vi "Calculate Particle Scores.vi"(7 "Pixel Value":i32=1, 8 "Limit Tests?":bool=TRUE, 9 "Aspect Fudge Factor":dbl=1.0, 10 "Sorted Data":dbl[][](array[numeric]), 11 "Image in":T2) -> (3 "Scores":T1(array[cluster]))   [LabVIEW 2015]
doc: "Calculate scores based on the particle measurements. Calculated scores are for aspect ratio, area to convex hull area, masking, and moment of inertia. These scores range between 0 and 100 and can be used to categorize particles as targets and non-targets. The fudge factor compensates for camera modes that do not give square pixels."
uses:
  <vilib>/vision/Image Controls.llb/IMAQ Image.ctl
  <vilib>/vision/NI_Vision_Development_Module.lvlib
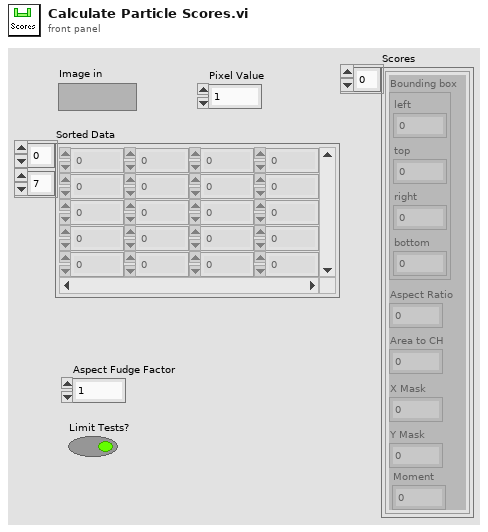
[diagram p1: front panel]
types:
  T1 = cluster{"Bounding box":cluster{"left":dbl, "top":dbl, "right":dbl, "bottom":dbl}, "Aspect Ratio":dbl, "Area to CH":dbl, "X Mask":dbl, "Y Mask":dbl, "Moment":dbl}[]
  T2 = typedef "IMAQ Image.ctl" = refnum<image>
  T3 = cluster{"[0]":dbl, "[1]":dbl, "[2]":dbl, "[3]":dbl}
  T4 = cluster{cluster{"[0]":dbl, "[1]":dbl, "[2]":dbl, "[3]":dbl}, "Aspect Ratio Score":dbl, "Score":dbl, "X Score":dbl, "Y Score":dbl, "Score":dbl}
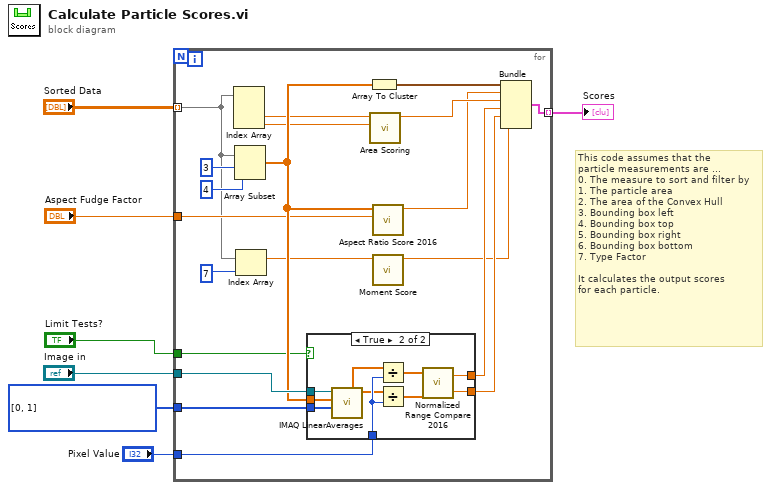
[diagram p0: block diagram]
diagram:
  w5 = i32[] [0, 1] items=["X Axis Averages", "Y Axis Averages", "X + Y Axis Averages", "X - Y Axis Averages"] ("Averages")
  # "This code assumes that the\nparticle measurements are ...\n0. The measure to sort and filter by\n1. The particle area\n2. The area of the Convex Hull\n3. Bounding box left\n4. Bounding box top\n5. Bounding box right\n6. Bounding box bottom\n7. Type Factor\n\nIt calculates the output scores\nfor each particle."
  n1 = for {
    tunnel: "Image in" -> [w23]
    tunnel: "Sorted Data" -> [w11] mode=indexing
    tunnel: [w25] -> w6 mode=indexing
    tunnel: w5 -> [w18]
    tunnel: "Pixel Value" -> [w16]
    tunnel: "Aspect Fudge Factor" -> [w13]
    tunnel: "Limit Tests?" -> [w12]
    n2 = Index Array(array=w11) -> (element #2=w15:dbl, element #3=w14:dbl)  [unwired: 3 in, 1 out]
    n3 = Array Subset(array=w11, index=3, length=4) -> (w17:dbl[])
    n4 = Index Array(array=w11, index=7 ("length")) -> (element=w9:dbl)
    n5 = case shown="True" w12 {
      tunnel: w23 -> [_ w37]
      tunnel: [_ w36] -> w20
      tunnel: [_ w35] -> w19
      tunnel: w18 -> [_ w34]
      tunnel: w17 -> [_ w33]
      tunnel: w16 -> [_ w32]
      frame False {
      }
      frame True {
        n6 = call "IMAQ LinearAverages"("Averages"=w34, "Optional Rectangle"=w33, "Image Src"=w37) -> ("Y Axis Averages"=w30:sgl[], "X Axis Averages"=w31:sgl[])  [unwired: 4 in, 3 out]
        n7 = Divide(x=w31, y=w32) -> (x/y=w29:sgl[])
        n8 = Divide(x=w30, y=w32) -> (x/y=w28:sgl[])
        n9 = call "Normalized Range Compare 2016.vi"("Y Averages"=w28, "X Averages"=w29) -> ("Y Score"=w35:dbl, "X Score"=w36:dbl)
      }
    }
    n10 = Array To Cluster(array=w17) -> (cluster=w22:T3)
    n11 = call "Area Scoring.vi"("Convex Hull Area"=w14, "Area"=w15) -> ("Score"=w24:dbl)  [unwired: 9 in]
    n12 = call "Aspect Ratio Score 2016.vi"("Aspect Fudge Factor"=w13, "Rectangle Array ltrb"=w17) -> ("Aspect Ratio Score"=w21:dbl)  [unwired: 9 in]
    n13 = call "Moment Score.vi"("Moment Factor"=w9) -> ("Score"=w8:dbl)  [unwired: 10 in]
    n14 = Bundle(w22, "Aspect Ratio Score"=w21, "Score"=w24, "X Score"=w20, "Y Score"=w19, "Score"=w8) -> (w25:T4)  [unwired: 1 in]
  }
  "Scores" <- w6
